vi "ErrorToResistance.vi"(2 "PID reading":dbl format="%#_13g", 3 "Bridge settings":T1) -> (0 "Voltage / V":dbl, 1 "Resistance / Ohms":dbl=25.0 format="%0.2f")   [LabVIEW 2014]
uses:
  controls/BridgeSettings.ctl
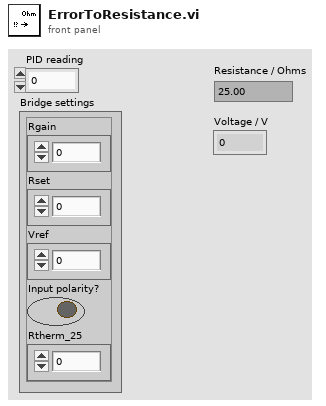
[diagram p1: front panel]
types:
  T1 = typedef "BridgeSettings.ctl" = cluster{"Rgain":dbl, "Rset":dbl, "Vref":dbl, "Input polarity?":bool, "Rtherm_25":dbl}
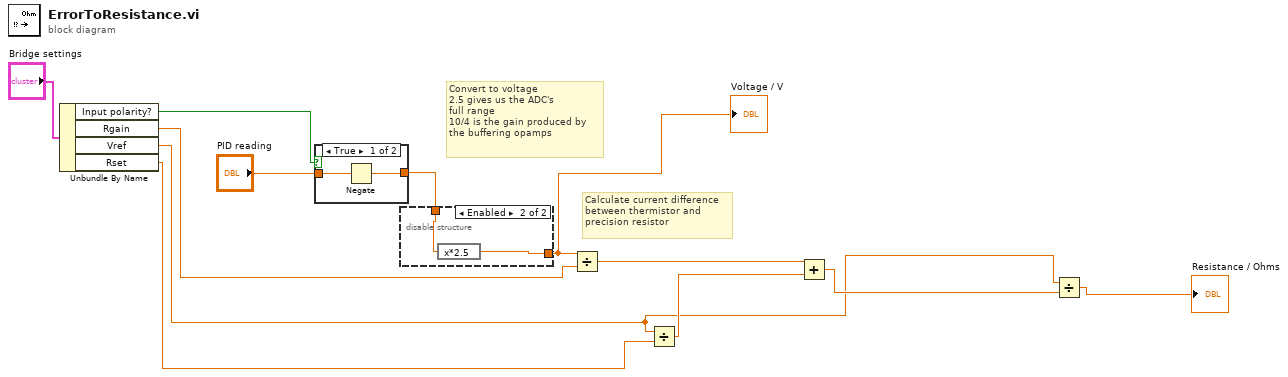
[diagram p0: block diagram]
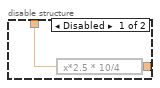
[diagram p3: hidden frame]
diagram:
  # "Calculate current difference\nbetween thermistor and\nprecision resistor"
  # "Convert to voltage\n2.5 gives us the ADC's \nfull range\n10/4 is the gain produced by \nthe buffering opamps"
  n1 = Unbundle By Name("Bridge settings") -> ("Input polarity?"=w5:bool, "Rgain"=w4:dbl, "Vref"=w3:dbl, "Rset"=w2:dbl)
  n2 = case shown="True" w5 {
    tunnel: [w13 w15] -> w8
    tunnel: "PID reading" -> [w14 w15]
    frame True {
      n3 = Negate(x=w14) -> (-x=w13:dbl)
    }
    frame False {
    }
  }
  n4 = disable-structure shown="Enabled" {
    disable-tunnel: w8 -> [w17 w18]
    disable-tunnel: [w16 w19] -> w10
    frame Disabled {
      n5 = expression code="x*2.5 * 10/4"(w17) -> (w16:dbl)
    }
    frame Enabled {
      n6 = expression code="x*2.5"(w18) -> (w19:dbl)
    }
  }
  "Voltage / V" <- w10
  n7 = Divide(x=w10, y=w4) -> (x/y=w12:dbl)
  n8 = Divide(x=w3, y=w2) -> (x/y=w11:dbl)
  n9 = Add(x=w12, y=w11) -> (x+y=w7:dbl)
  n10 = Divide(x=w3, y=w7) -> (x/y=→"Resistance / Ohms":dbl)
